vi "pcbAlignment.vi"() -> ()   [LabVIEW 2015]
uses:
  GlobalPath.vi
  GlobalData.vi
  GlobalVi.vi
panel:
  out "appended path":path
  out "appended path":path
  out "Execution:State":T1(ring)
  out "rasnik program 2":bool
  out "Open Program 2":bool
  in  "Open Program 6":bool
  out "Mapping file":string
  in  "?":bool
  in  "visual 4":bool caption="Close the PCB gaps to not lose vacuum pressure"
  in  "Open Program 5":bool
  in  "Open Program 4":bool
  in  "Done with vacuum test?":bool
  in  "c-ccd 9":bool caption="Place the movement arch away from the table"
  in  "c-ccd 8":bool caption="Release the movement arch from the stiffback"
  in  "c-ccd 7":bool caption="Lower the stiffback on the table"
  in  "c-ccd 6":bool caption="Move the stiffback over the table"
  in  "Open Program 3":bool
  out "PanelName":string
  in  "rasnik program":bool
  in  "Done with PCB testing?":bool
  in  "Open Program":bool
  in  "c-ccd 4":bool caption="Remove the 10 reference pins"
  in  "visual 3":bool caption="Turn vacuum on for PCB blocking"
  in  "Done?":bool
  in  "visual 2":bool caption="Position the 10 reference pins for the PCB alignment"
  # "PCB alignment on table/stiffback"
  # "Vacuum testing"
  # "Open the pressure monitoring program and let it run on the background"
  # "and press \"Start\" to start the pressure recording"
  # "Check the PCB vacuum"
  # "choose the date and press ok to make sure the pressure levels are alright"
  # "Rasnik mask reading from C-CCDs"
  # "The PCB on the table/stiffback will be read through the appropriate vi program"
  # "Post-alignment"
  # "PCB testing"
  # "At this point, the PCB on the table/stiffback will be tested in the appropriate vi program"
  # "PCB MAPPING"
  # "IN CASE OF PCB QUALITY PROBLEMS:\n(only press if need of PCB substitution)"
  # "FRAME/COOLING BAR MAPPING"
  # "Loading the raw file to the database:\nGo to the Database, select the tab \"PCB\" and then for each PCB (cross-check the positions from the \"Position\" selection within each PCB tab) click on \"Load Raw\"\nand choose the appropritate file to load ---->\nClick on \"Add/Update Entry\""
  # "(If the database window is closed, then click here  -->                 and load the correct panel this way: Add>Add then from the list choose \"Readout\" and then Start\n                                                                                                                                                                                                                     Choose the correct ID and click \"Start building panel\")"
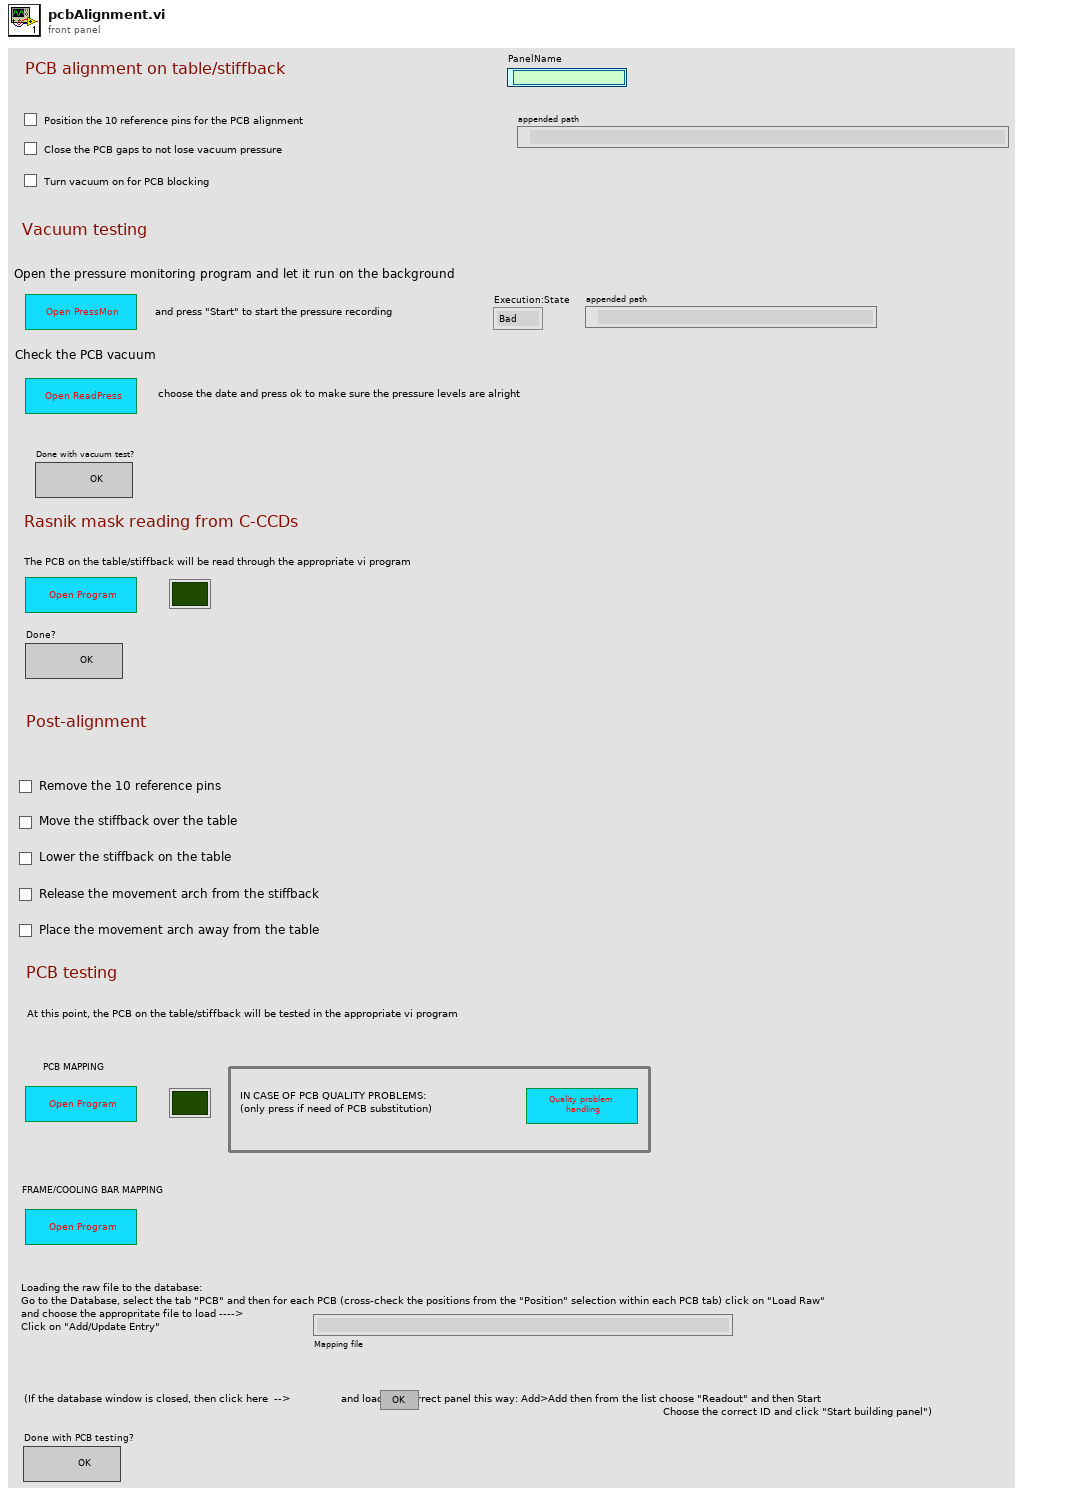
[diagram p1: front panel]
types:
  T1 = enum32{"Bad", "Idle", "Run top level", "Running"}
  T2 = enum16{"open", "replace", "create", "open or create", "replace or create", "replace or create with confirmation"}
  T3 = enum8{"Enabled", "Disabled", "Disabled and Grayed Out"}
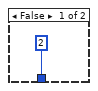
[diagram p4: hidden frame]
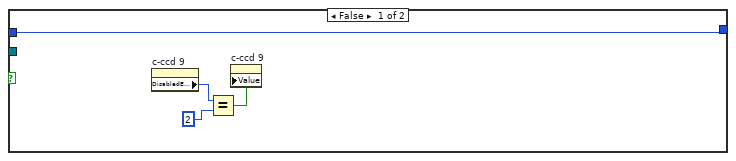
[diagram p8: hidden frame]
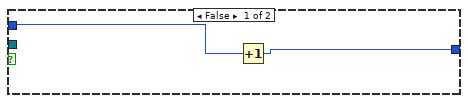
[diagram p9: hidden frame]
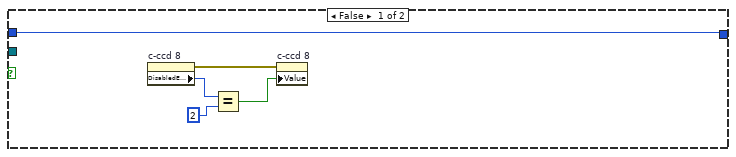
[diagram p10: hidden frame]
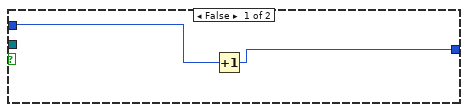
[diagram p11: hidden frame]
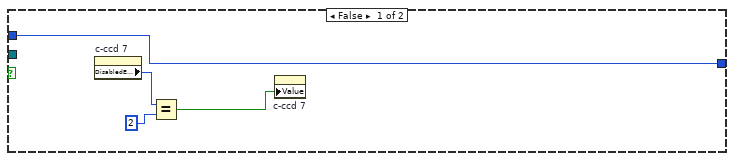
[diagram p12: hidden frame]
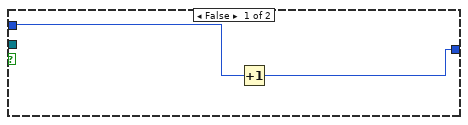
[diagram p13: hidden frame]
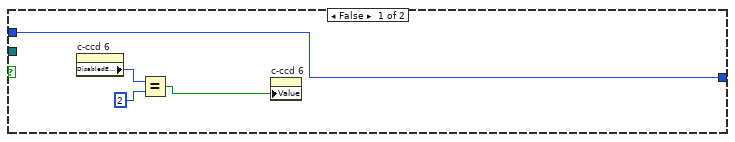
[diagram p14: hidden frame]
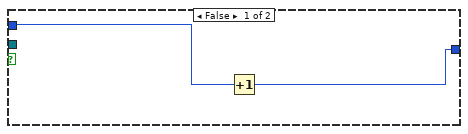
[diagram p15: hidden frame]
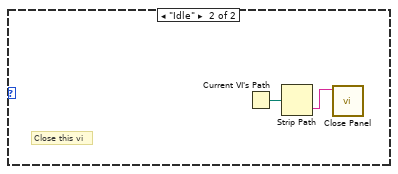
[diagram p19: hidden frame]
diagram:
  n1 = flat-sequence {
    tunnel: [w13] -> w10
    tunnel: [w12] -> w9
    tunnel: w10 -> [w73]
    tunnel: w9 -> [w72]
    tunnel: [w73] -> w8
    tunnel: [w72] -> w7
    tunnel: w8 -> [w411]
    tunnel: w7 -> [w410]
    tunnel: [w404] -> w6
    tunnel: [w409] -> w5
    tunnel: w6 -> [w513]
    tunnel: w5 -> [w524]
    tunnel: [w524] -> w4
    tunnel: [w512] -> w2
    tunnel: w4 -> [w539]
    tunnel: [w539] -> w3
    tunnel: w2 -> [w535]
    tunnel: [w534] -> w1
    tunnel: w3 -> [_]
    tunnel: w1 -> [_]
    frame #0 {
      n2 = flat-sequence {
        tunnel: [w26] -> w14
        tunnel: [w25] -> w11
        tunnel: w14 -> [w55]
        tunnel: [w54] -> w13
        tunnel: [w53] -> w12
        tunnel: w11 -> [w52]
        frame #0 {
          n3 = global read "GlobalData.vi" "PanelName"() -> (w20:string)
          n4 = global read "GlobalPath.vi" "LogFilesDir"() -> (w18:path)
          n5 = global read "GlobalData.vi" "Stage"() -> (w17:string)
          n6 = Empty String/Path?(string/path=w17) -> (empty?=w19:bool)
          n7 = Empty String/Path?(string/path=w20) -> (empty?=w21:bool)
          n8 = case shown="True" w19 {
            tunnel: w18 -> [_ w38]
            tunnel: [w32 w33] -> w16
            tunnel: w17 -> [w32 _]
            frame False {
            }
            frame True {
              n9 = Build Path(base path=w38, name or relative path="Stage.log") -> (appended path=w37:path)
              n10 = Open/Create/Replace File(file path (use dialog)=w37) -> (refnum out=w34:refnum<file>, error out=w35:errorcluster)  [unwired: 5 in, 1 out]
              n11 = Read from Text File(file (use dialog)=w34, error in=w35) -> (text=w33:string)  [unwired: 2 in, 3 out]
              n12 = global write "GlobalData.vi" "Stage"(w33) -> ()
            }
          }
          n13 = case shown="True" w21 {
            tunnel: w18 -> [_ w45]
            tunnel: [w39 w40] -> w15
            tunnel: w20 -> [w39 _]
            frame False {
            }
            frame True {
              n14 = Build Path(base path=w45, name or relative path="PanelName.log") -> (appended path=w44:path)
              n15 = Open/Create/Replace File(file path (use dialog)=w44) -> (refnum out=w41:refnum<file>, error out=w42:errorcluster)  [unwired: 5 in, 1 out]
              n16 = Read from Text File(file (use dialog)=w41, error in=w42) -> (text=w40:string)  [unwired: 2 in, 3 out]
              n17 = global write "GlobalData.vi" "PanelName"(w40) -> ()
            }
          }
          "PanelName" <- w15
          n18 = Equal?(x=w16, y="Stiffback") -> (x = y?=w23:bool)
          n19 = Build Path(base path=w18, name or relative path=w15) -> (appended path=w31:path)
          "appended path" <- w31
          n20 = case shown="True" w23 {
            tunnel: [2 0] -> w22
            frame False {
            }
            frame True {
            }
          }
          n21 = property on="c-ccd 6" class="Bool (strict)"("DisabledEnum"=w22) -> ()  [unwired: 2 in, 2 out]
          n22 = property on="c-ccd 8" class="Bool (strict)"("DisabledEnum"=w22) -> ()  [unwired: 2 in, 2 out]
          n23 = property on="c-ccd 9" class="Bool (strict)"("DisabledEnum"=w22) -> ()  [unwired: 2 in, 2 out]
          n24 = property on="c-ccd 7" class="Bool (strict)"("DisabledEnum"=w22) -> ()  [unwired: 2 in, 2 out]
          n25 = Open/Create/Replace File(file path (use dialog)=w31, operation (0:open)=T2."open") -> (refnum out=w28:refnum<file>, error out=w27:errorcluster)  [unwired: 4 in, 1 out]
          n26 = Set File Position(refnum=w28, from (0:start)=enum16{"start", "end", "current"}."end", error in=w27) -> (refnum out=w26:refnum<file>, error out=w25:errorcluster)  [unwired: 1 in]
        }
        frame #1 {
          w48 = "\r"
          n27 = Get Date/Time In Seconds() -> (seconds since 1Jan1904=w51:timestamp)
          n28 = global read "GlobalData.vi" "Stage"() -> (w50:string)
          n29 = Format Date/Time String(seconds (now)=w51) -> (date/time string=w57:string)  [unwired: 2 in]
          n30 = Concatenate Strings(w48, w57, "\t", " PCB ALIGNMENT ", w50, ": ", w48) -> (w56:string)
          n31 = Write to Text File(file (use dialog)=w55, text=w56, error in=w52) -> (refnum out=w54:refnum<file>, error out=w53:errorcluster)  [unwired: 1 in, 1 out]
        }
      }
    }
    frame #1 {
      n32 = while {
        tunnel: w73 -> [w81]
        shift-right: [w132] -> _
        shift-left: 0 -> [w130]
        shift-right: [w127] -> _
        shift-left: 0 -> [w123]
        shift-right: [w114] -> _
        shift-left: 0 -> [w119]
        shift-right: [w115] -> _
        shift-left: 0 -> [w116]
        shift-right: [w109] -> _
        shift-left: 0 -> [w110]
        shift-right: [w104] -> _
        shift-left: 0 -> [w106]
        shift-right: [w92] -> _
        shift-left: 0 -> [w99]
        shift-right: [w93] -> _
        shift-left: 0 -> [w98]
        shift-right: [w94] -> _
        shift-left: 0 -> [w97]
        shift-right: [w95] -> _
        shift-left: 0 -> [w96]
        shift-right: [w84] -> _
        shift-left: 0 -> [w85]
        shift-right: [w79] -> _
        shift-left: 0 -> [w82]
        stop <- w134 stop-if-true
        n33 = Compound Arithmetic op=AND("visual 2", "visual 3", "Open Program 4", "Done?", "c-ccd 4", "visual 4", "Open Program 6", "c-ccd 6", "c-ccd 7", "c-ccd 8", "c-ccd 9") -> (w134:bool)
        n34 = Equal To 0?(x=w82) -> (x = 0?=w83:bool)
        n35 = Equal To 0?(x=w119) -> (x = 0?=w122:bool)
        n36 = Equal To 0?(x=w106) -> (x = 0?=w108:bool)
        n37 = Equal To 0?(x=w99) -> (x = 0?=w103:bool)
        n38 = Equal To 0?(x=w97) -> (x = 0?=w101:bool)
        n39 = Equal To 0?(x=w96) -> (x = 0?=w100:bool)
        n40 = Equal To 0?(x=w130) -> (x = 0?=w129:bool)
        n41 = Equal To 0?(x=w98) -> (x = 0?=w102:bool)
        n42 = Equal To 0?(x=w110) -> (x = 0?=w113:bool)
        n43 = Equal To 0?(x=w116) -> (x = 0?=w118:bool)
        n44 = Equal To 0?(x=w123) -> (x = 0?=w126:bool)
        n45 = Wait (ms)(milliseconds to wait=u32 50) -> ()  [unwired: 1 out]
        n46 = And(x="Open Program 6", y=w83) -> (x .and. y?=w80:bool)
        n47 = And(x="rasnik program", y=w122) -> (x .and. y?=w120:bool)
        n48 = And(x="c-ccd 4", y=w108) -> (x .and. y?=w107:bool)
        n49 = And(x="c-ccd 6", y=w103) -> (x .and. y?=w88:bool)
        n50 = And(x="c-ccd 8", y=w101) -> (x .and. y?=w90:bool)
        n51 = And(x="c-ccd 9", y=w100) -> (x .and. y?=w91:bool)
        n52 = And(x="visual 2", y=w129) -> (x .and. y?=w128:bool)
        n53 = And(x="c-ccd 7", y=w102) -> (x .and. y?=w89:bool)
        n54 = And(x="Done?", y=w113) -> (x .and. y?=w111:bool)
        n55 = And(x="Open Program 4", y=w118) -> (x .and. y?=w117:bool)
        n56 = And(x="visual 3", y=w126) -> (x .and. y?=w124:bool)
        n57 = case shown="True" w111 {
          tunnel: w81 -> [_ w290]
          tunnel: [w286 w289] -> w109
          tunnel: w110 -> [w286 w288]
          frame False {
          }
          frame True {
            n58 = flat-sequence {
              tunnel: w290 -> [w293]
              tunnel: [w292] -> w291
              tunnel: w288 -> [w292]
              tunnel: w291 -> [w297]
              tunnel: [w298] -> w287
              tunnel: [w299] -> w289
              tunnel: w287 -> [w299]
              frame #0 {
                n59 = Concatenate Strings("Done with Rasmask reading", "\r") -> (w296:string)
                n60 = Write to Text File(file (use dialog)=w293, text=w296) -> ()  [unwired: 2 in, 3 out]
              }
              frame #1 {
                n61 = Increment(x=w297) -> (x+1=w298:i32)
              }
              frame #2 {
                n62 = while {
                  stop <- TRUE stop-if-true
                  n63 = property on="Open Program 3" class="Bool (strict)"() -> ("Value"=w301:bool)  [unwired: 2 in, 2 out]
                  n64 = Wait (ms)(milliseconds to wait=10000) -> ()  [unwired: 1 out]
                  n65 = Equal?(x=w301, y=TRUE) -> (x = y?=w303:bool)
                  n66 = case shown="True" w303 {
                    frame False {
                    }
                    frame True {
                      # "Automatically open the QualityProblemHandling.vi and close the current vi once done"
                      n67 = global read "GlobalPath.vi" "ViDir"() -> (w307:path)
                      n68 = call "OpenNRun.vi"("VI name"="QualityProblemHandling.vi", "ViDirPath"=w307) -> ("Execution:State"=w306:T1)
                      n69 = case shown="\"Bad\", Default" w306 {
                        frame "Bad", Default {
                          n70 = flat-sequence {
                            tunnel: [w309] -> w308
                            tunnel: w308 -> [w312]
                            frame #0 {
                              n71 = call "Display Message to User5"() -> ("error out"=w309:errorcluster)  [unwired: 10 in, 1 out]
                            }
                            frame #1 {
                              n72 = Current VI's Path() -> (path=w310:path)
                              n73 = Open VI Reference(vi path=w310, error in (no error)=w312) -> (vi reference=w315:refnum<vi>, error out=w314:errorcluster)  [unwired: 4 in]
                              n74 = global read "GlobalPath.vi" "ViDir"() -> (w311:path)
                              n75 = property class="VI"(reference=w315, error in=w314) -> ("Name"=w313:string)  [unwired: 2 out]
                              n76 = call "OpenNRun.vi"("VI name"=w313, "ViDirPath"=w311) -> ()  [unwired: 1 out]
                            }
                          }
                        }
                        frame "Idle" {
                          # "Close this vi"
                          n77 = Current VI's Path() -> (path=w317:path)
                          n78 = Strip Path(path=w317) -> (name=w316:string)  [unwired: 1 out]
                          n79 = call <vilib>:"Close Panel.vi"("VI name"=w316) -> ()  [unwired: 10 in, 1 out]
                        }
                      }
                    }
                  }
                }
              }
            }
          }
        }
        n80 = case shown="True" w80 {
          tunnel: w81 -> [_ w143]
          tunnel: [w135 w142] -> w79
          tunnel: w82 -> [w135 w141]
          frame False {
          }
          frame True {
            n81 = flat-sequence {
              tunnel: w143 -> [w145]
              tunnel: [w146] -> w144
              tunnel: w141 -> [w146]
              tunnel: [w145] -> w138
              tunnel: w144 -> [w154]
              tunnel: [w155] -> w140
              tunnel: w138 -> [w153]
              tunnel: [w153] -> w136
              tunnel: w140 -> [w162]
              tunnel: [w162] -> w139
              tunnel: [w161] -> w137
              tunnel: w136 -> [w161]
              tunnel: [w168] -> w142
              tunnel: w139 -> [w168]
              tunnel: w137 -> [w164]
              frame #0 {
                n82 = Concatenate Strings("Calling readpress.vi", "\r") -> (w149:string)
                n83 = Write to Text File(file (use dialog)=w145, text=w149) -> ()  [unwired: 2 in, 3 out]
              }
              frame #1 {
                n84 = global read "GlobalPath.vi" "ViDir"() -> (w152:path)
                n85 = Increment(x=w154) -> (x+1=w155:i32)
                n86 = call "OpenNRun.vi"("VI name"="readPress.vi", "ViDirPath"=w152) -> ("Execution:State"=w150:T1)
                n87 = case shown="\"Bad\", Default" w150 {
                  frame "Bad", Default {
                    n88 = flat-sequence {
                      frame #0 {
                        n89 = call "Display Message to User9"() -> ()  [unwired: 10 in, 2 out]
                      }
                      frame #1 {
                        n90 = Current VI's Path() -> (path=w156:path)
                        n91 = Open VI Reference(vi path=w156) -> (vi reference=w160:refnum<vi>, error out=w159:errorcluster)  [unwired: 5 in]
                        n92 = global read "GlobalPath.vi" "ViDir"() -> (w158:path)
                        n93 = property class="VI"(reference=w160, error in=w159) -> ("Name"=w157:string)  [unwired: 2 out]
                        n94 = call "OpenNRun.vi"("VI name"=w157, "ViDirPath"=w158) -> ()  [unwired: 1 out]
                      }
                    }
                  }
                  frame "Idle" {
                  }
                }
              }
              frame #2 {
                n95 = while {
                  stop <- "Done with vacuum test?" stop-if-true
                }
              }
              frame #3 {
                n96 = Concatenate Strings("Done with reading pressure", "\r") -> (w167:string)
                n97 = Write to Text File(file (use dialog)=w164, text=w167) -> ()  [unwired: 2 in, 3 out]
              }
            }
          }
        }
        n98 = case shown="True" w88 {
          tunnel: w99 -> [w251 w260]
          tunnel: w81 -> [_ w259]
          tunnel: [w251 w258] -> w92
          frame False {
            n99 = property on="c-ccd 6" class="Bool (strict)"() -> ("DisabledEnum"=w253:T3)  [unwired: 2 in, 2 out]
            n100 = Equal?(x=w253, y=2) -> (x = y?=w252:bool)
            n101 = property on="c-ccd 6" class="Bool (strict)"("Value"=w252) -> ()  [unwired: 2 in, 2 out]
          }
          frame True {
            n102 = property on="c-ccd 6" class="Bool (strict)"() -> ("DisabledEnum"=w256:T3)  [unwired: 2 in, 2 out]
            n103 = Equal?(x=w256, y=0) -> (x = y?=w255:bool)
            n104 = case shown="True" w255 {
              tunnel: w259 -> [_ w265]
              tunnel: [w261 w264] -> w258
              tunnel: w260 -> [w262 w263]
              frame False {
                n105 = Increment(x=w262) -> (x+1=w261:i32)
              }
              frame True {
                n106 = flat-sequence {
                  tunnel: w265 -> [w268]
                  tunnel: [w267] -> w266
                  tunnel: w263 -> [w267]
                  tunnel: w266 -> [w272]
                  tunnel: [w273] -> w264
                  frame #0 {
                    n107 = Concatenate Strings("Stiffback moved over table", "\r") -> (w271:string)
                    n108 = Write to Text File(file (use dialog)=w268, text=w271) -> ()  [unwired: 2 in, 3 out]
                  }
                  frame #1 {
                    n109 = Increment(x=w272) -> (x+1=w273:i32)
                  }
                }
              }
            }
          }
        }
        n110 = case shown="True" w89 {
          tunnel: w81 -> [_ w237]
          tunnel: w98 -> [w228 w236]
          tunnel: [w228 w235] -> w93
          frame False {
            n111 = property on="c-ccd 7" class="Bool (strict)"() -> ("DisabledEnum"=w230:T3)  [unwired: 2 in, 2 out]
            n112 = Equal?(x=w230, y=2) -> (x = y?=w229:bool)
            n113 = property on="c-ccd 7" class="Bool (strict)"("Value"=w229) -> ()  [unwired: 2 in, 2 out]
          }
          frame True {
            n114 = property on="c-ccd 7" class="Bool (strict)"() -> ("DisabledEnum"=w233:T3)  [unwired: 2 in, 2 out]
            n115 = Equal?(x=w233, y=0) -> (x = y?=w232:bool)
            n116 = case shown="True" w232 {
              tunnel: w237 -> [_ w242]
              tunnel: [w238 w241] -> w235
              tunnel: w236 -> [w239 w240]
              frame False {
                n117 = Increment(x=w239) -> (x+1=w238:i32)
              }
              frame True {
                n118 = flat-sequence {
                  tunnel: w242 -> [w245]
                  tunnel: [w244] -> w243
                  tunnel: w240 -> [w244]
                  tunnel: w243 -> [w249]
                  tunnel: [w250] -> w241
                  frame #0 {
                    n119 = Concatenate Strings("Stiffback lowered on table", "\r") -> (w248:string)
                    n120 = Write to Text File(file (use dialog)=w245, text=w248) -> ()  [unwired: 2 in, 3 out]
                  }
                  frame #1 {
                    n121 = Increment(x=w249) -> (x+1=w250:i32)
                  }
                }
              }
            }
          }
        }
        n122 = case shown="True" w90 {
          tunnel: w81 -> [_ w214]
          tunnel: w97 -> [w204 w213]
          tunnel: [w204 w212] -> w94
          frame False {
            n123 = property on="c-ccd 8" class="Bool (strict)"() -> (error out=w208:errorcluster, "DisabledEnum"=w206:T3)  [unwired: 2 in, 1 out]
            n124 = Equal?(x=w206, y=2) -> (x = y?=w205:bool)
            n125 = property on="c-ccd 8" class="Bool (strict)"(error in=w208, "Value"=w205) -> ()  [unwired: 1 in, 2 out]
          }
          frame True {
            n126 = property on="c-ccd 8" class="Bool (strict)"() -> ("DisabledEnum"=w210:T3)  [unwired: 2 in, 2 out]
            n127 = Equal?(x=w210, y=0) -> (x = y?=w209:bool)
            n128 = case shown="True" w209 {
              tunnel: w214 -> [_ w219]
              tunnel: [w215 w218] -> w212
              tunnel: w213 -> [w216 w217]
              frame False {
                n129 = Increment(x=w216) -> (x+1=w215:i32)
              }
              frame True {
                n130 = flat-sequence {
                  tunnel: w219 -> [w222]
                  tunnel: [w221] -> w220
                  tunnel: w217 -> [w221]
                  tunnel: w220 -> [w226]
                  tunnel: [w227] -> w218
                  frame #0 {
                    n131 = Concatenate Strings("Arch released", "\r") -> (w225:string)
                    n132 = Write to Text File(file (use dialog)=w222, text=w225) -> ()  [unwired: 2 in, 3 out]
                  }
                  frame #1 {
                    n133 = Increment(x=w226) -> (x+1=w227:i32)
                  }
                }
              }
            }
          }
        }
        n134 = case shown="True" w91 {
          tunnel: w81 -> [_ w186]
          tunnel: w96 -> [w181 w187]
          tunnel: [w181 w185] -> w95
          frame False {
            n135 = property on="c-ccd 9" class="Bool (strict)"() -> ("DisabledEnum"=w183:T3)  [unwired: 2 in, 2 out]
            n136 = Equal?(x=w183, y=2) -> (x = y?=w182:bool)
            n137 = property on="c-ccd 9" class="Bool (strict)"("Value"=w182) -> ()  [unwired: 2 in, 2 out]
          }
          frame True {
            n138 = property on="c-ccd 9" class="Bool (strict)"() -> ("DisabledEnum"=w189:T3)  [unwired: 2 in, 2 out]
            n139 = Equal?(x=w189, y=0) -> (x = y?=w188:bool)
            n140 = case shown="True" w188 {
              tunnel: w186 -> [_ w195]
              tunnel: [w191 w194] -> w185
              tunnel: w187 -> [w192 w193]
              frame False {
                n141 = Increment(x=w192) -> (x+1=w191:i32)
              }
              frame True {
                n142 = flat-sequence {
                  tunnel: w195 -> [w198]
                  tunnel: [w197] -> w196
                  tunnel: w193 -> [w197]
                  tunnel: w196 -> [w202]
                  tunnel: [w203] -> w194
                  frame #0 {
                    n143 = Concatenate Strings("Arch moved away", "\r") -> (w201:string)
                    n144 = Write to Text File(file (use dialog)=w198, text=w201) -> ()  [unwired: 2 in, 3 out]
                  }
                  frame #1 {
                    n145 = Increment(x=w202) -> (x+1=w203:i32)
                  }
                }
              }
            }
          }
        }
        n146 = case shown="True" w117 {
          tunnel: w81 -> [_ w326]
          tunnel: [w318 w325] -> w115
          tunnel: w116 -> [w318 w324]
          frame False {
          }
          frame True {
            n147 = flat-sequence {
              tunnel: w326 -> [w328]
              tunnel: [w329] -> w327
              tunnel: w324 -> [w329]
              tunnel: [w328] -> w321
              tunnel: w327 -> [w341]
              tunnel: [w342] -> w323
              tunnel: w321 -> [w340]
              tunnel: [w340] -> w319
              tunnel: w323 -> [w352]
              tunnel: [w352] -> w322
              tunnel: [w351] -> w320
              tunnel: w319 -> [w351]
              tunnel: [w357] -> w325
              tunnel: w322 -> [w357]
              tunnel: w320 -> [w353]
              frame #0 {
                n148 = Concatenate Strings("Calling pressmon.vi", "\r") -> (w332:string)
                n149 = Write to Text File(file (use dialog)=w328, text=w332) -> ()  [unwired: 2 in, 3 out]
              }
              frame #1 {
                w336 = "pressmon.vi"
                n150 = global read "GlobalPath.vi" "ViDir"() -> (w334:path)
                n151 = Increment(x=w341) -> (x+1=w342:i32)
                n152 = Build Path(base path=path "/home/atlas/Micromegas/interface" ("ViDir"), name or relative path=w336) -> (appended path=w337:path)
                "appended path" <- w337
                n153 = Open VI Reference(vi path=w337) -> (vi reference=w338:refnum<vi>, error out=w339:errorcluster)  [unwired: 5 in]
                n154 = property class="VI"(reference=w338, error in=w339) -> ("Exec.State"=w335:T1)  [unwired: 2 out]
                "Execution:State" <- w335
                n155 = case shown="\"Bad\", Default" w335 {
                  tunnel: w336 -> [_ w345 _ _]
                  tunnel: w334 -> [_ w343 _ _]
                  frame "Bad", Default {
                  }
                  frame "Idle" {
                    n156 = call "OpenNRun.vi"("VI name"=w345, "ViDirPath"=w343) -> ("Execution:State"=w344:T1)
                    n157 = case shown="\"Bad\", Default" w344 {
                      frame "Bad", Default {
                        n158 = flat-sequence {
                          frame #0 {
                            n159 = call "Display Message to User6"() -> ()  [unwired: 10 in, 2 out]
                          }
                          frame #1 {
                            n160 = Current VI's Path() -> (path=w346:path)
                            n161 = Open VI Reference(vi path=w346) -> (vi reference=w350:refnum<vi>, error out=w349:errorcluster)  [unwired: 5 in]
                            n162 = global read "GlobalPath.vi" "ViDir"() -> (w348:path)
                            n163 = property class="VI"(reference=w350, error in=w349) -> ("Name"=w347:string)  [unwired: 2 out]
                            n164 = call "OpenNRun.vi"("VI name"=w347, "ViDirPath"=w348) -> ()  [unwired: 1 out]
                          }
                        }
                      }
                      frame "Idle" {
                      }
                    }
                  }
                  frame "Run top level" {
                  }
                  frame "Running" {
                  }
                }
              }
              frame #2 {
              }
              frame #3 {
                n165 = Concatenate Strings("Done with pressure monitoring", "\r") -> (w356:string)
                n166 = Write to Text File(file (use dialog)=w353, text=w356) -> ()  [unwired: 2 in, 3 out]
              }
            }
          }
        }
        n167 = case shown="True" w107 {
          tunnel: w81 -> [_ w277]
          tunnel: [w274 w276] -> w104
          tunnel: w106 -> [w274 w275]
          frame False {
          }
          frame True {
            n168 = flat-sequence {
              tunnel: w277 -> [w280]
              tunnel: [w279] -> w278
              tunnel: w275 -> [w279]
              tunnel: w278 -> [w284]
              tunnel: [w285] -> w276
              frame #0 {
                n169 = Concatenate Strings("Reference pins removed", "\r") -> (w283:string)
                n170 = Write to Text File(file (use dialog)=w280, text=w283) -> ()  [unwired: 2 in, 3 out]
              }
              frame #1 {
                n171 = Increment(x=w284) -> (x+1=w285:i32)
              }
            }
          }
        }
        n172 = case shown="True" w120 {
          tunnel: w81 -> [_ w361]
          tunnel: [w358 w359] -> w114
          tunnel: w119 -> [w358 w360]
          frame False {
          }
          frame True {
            n173 = flat-sequence {
              tunnel: w361 -> [w364]
              tunnel: [w363] -> w362
              tunnel: w360 -> [w363]
              tunnel: w362 -> [w371]
              tunnel: [w372] -> w359
              frame #0 {
                n174 = Concatenate Strings("Calling Rasnik.vi", "\r") -> (w367:string)
                n175 = Write to Text File(file (use dialog)=w364, text=w367) -> ()  [unwired: 2 in, 3 out]
              }
              frame #1 {
                n176 = global read "GlobalPath.vi" "ViDir"() -> (w368:path)
                n177 = Increment(x=w371) -> (x+1=w372:i32)
                n178 = call "OpenNRun.vi"("VI name"="Rasnik.vi", "ViDirPath"=w368) -> ("Execution:State"=w369:T1)
                n179 = case shown="\"Bad\", Default" w369 {
                  frame "Bad", Default {
                    n180 = flat-sequence {
                      frame #0 {
                        n181 = call "Display Message to User3"() -> ()  [unwired: 10 in, 2 out]
                      }
                      frame #1 {
                        n182 = Current VI's Path() -> (path=w373:path)
                        n183 = Open VI Reference(vi path=w373) -> (vi reference=w377:refnum<vi>, error out=w376:errorcluster)  [unwired: 5 in]
                        n184 = global read "GlobalPath.vi" "ViDir"() -> (w375:path)
                        n185 = property class="VI"(reference=w377, error in=w376) -> ("Name"=w374:string)  [unwired: 2 out]
                        n186 = call "OpenNRun.vi"("VI name"=w374, "ViDirPath"=w375) -> ()  [unwired: 1 out]
                      }
                    }
                  }
                  frame "Idle" {
                  }
                }
              }
            }
          }
        }
        n187 = case shown="True" w128 {
          tunnel: w81 -> [_ w394]
          tunnel: w130 -> [w390 w393]
          tunnel: [w390 w391] -> w132
          frame False {
          }
          frame True {
            n188 = flat-sequence {
              tunnel: w394 -> [w396]
              tunnel: w393 -> [w395]
              tunnel: [w395] -> w392
              tunnel: w392 -> [w401]
              tunnel: [w400] -> w391
              frame #0 {
                n189 = Concatenate Strings("10 reference pins positioned", "\r") -> (w399:string)
                n190 = Write to Text File(file (use dialog)=w396, text=w399) -> ()  [unwired: 2 in, 3 out]
              }
              frame #1 {
                n191 = Increment(x=w401) -> (x+1=w400:i32)
              }
            }
          }
        }
        n192 = case shown="True" "visual 4" {
          tunnel: w81 -> [_ w172]
          tunnel: [w169 w171] -> w84
          tunnel: w85 -> [w169 w170]
          frame False {
          }
          frame True {
            n193 = flat-sequence {
              tunnel: w172 -> [w175]
              tunnel: [w174] -> w173
              tunnel: w170 -> [w174]
              tunnel: w173 -> [w179]
              tunnel: [w180] -> w171
              frame #0 {
                n194 = Concatenate Strings("Closing gaps", "\r") -> (w178:string)
                n195 = Write to Text File(file (use dialog)=w175, text=w178) -> ()  [unwired: 2 in, 3 out]
              }
              frame #1 {
                n196 = Increment(x=w179) -> (x+1=w180:i32)
              }
            }
          }
        }
        n197 = case shown="True" w124 {
          tunnel: w81 -> [_ w381]
          tunnel: [w378 w380] -> w127
          tunnel: w123 -> [w378 w379]
          frame False {
          }
          frame True {
            n198 = flat-sequence {
              tunnel: w381 -> [w384]
              tunnel: [w383] -> w382
              tunnel: w379 -> [w383]
              tunnel: w382 -> [w388]
              tunnel: [w389] -> w380
              frame #0 {
                n199 = Concatenate Strings("Vacuum turned on for blocking", "\r") -> (w387:string)
                n200 = Write to Text File(file (use dialog)=w384, text=w387) -> ()  [unwired: 2 in, 3 out]
              }
              frame #1 {
                n201 = Increment(x=w388) -> (x+1=w389:i32)
              }
            }
          }
        }
        "rasnik program 2" <- "rasnik program"
      }
    }
    frame #2 {
      # "PCB testing"
      n202 = while {
        shift-right: [w436] -> w403
        shift-left: w410 -> [w435]
        stop <- "Open Program" stop-if-true
        n203 = case shown="True" "Open Program" {
          tunnel: [w437 w439] -> w436
          tunnel: w435 -> [w437 w442]
          frame False {
          }
          frame True {
            n204 = flat-sequence {
              tunnel: w442 -> [w444]
              tunnel: [w443] -> w438
              tunnel: [w463] -> w441
              tunnel: [w462] -> w440
              tunnel: w438 -> [w461]
              tunnel: w441 -> [w469]
              tunnel: w440 -> [w468]
              tunnel: [w467] -> w439
              frame #0 {
                n205 = global read "GlobalPath.vi" "ViDir"() -> (w447:path)
                n206 = call "OpenNRun.vi"("VI name"="map_trap_switch.vi", "ViDirPath"=w447) -> ("Execution:State"=w446:T1)
                n207 = case shown="\"Bad\", Default" w446 {
                  tunnel: [w450 w460] -> w443
                  tunnel: w444 -> [w449 w460]
                  frame "Bad", Default {
                    n208 = flat-sequence {
                      tunnel: w449 -> [w452]
                      tunnel: [w451] -> w448
                      tunnel: [w455] -> w450
                      tunnel: w448 -> [w453]
                      frame #0 {
                        n209 = call "Display Message to User"("error in (no error)"=w452) -> ("error out"=w451:errorcluster)  [unwired: 9 in, 1 out]
                      }
                      frame #1 {
                        n210 = Current VI's Path() -> (path=w454:path)
                        n211 = Open VI Reference(vi path=w454, error in (no error)=w453) -> (vi reference=w459:refnum<vi>, error out=w458:errorcluster)  [unwired: 4 in]
                        n212 = global read "GlobalPath.vi" "ViDir"() -> (w457:path)
                        n213 = property class="VI"(reference=w459, error in=w458) -> (error out=w455:errorcluster, "Name"=w456:string)  [unwired: 1 out]
                        n214 = call "OpenNRun.vi"("VI name"=w456, "ViDirPath"=w457) -> ()  [unwired: 1 out]
                      }
                    }
                  }
                  frame "Idle" {
                  }
                }
              }
              frame #1 {
                n215 = Open/Create/Replace File(file path (use dialog)=path "/home/atlas/Micromegas/M05Data/mapping/map_trap_filename.txt", error in=w461, operation (0:open)=T2."open") -> (refnum out=w463:refnum<file>, error out=w462:errorcluster)  [unwired: 3 in, 1 out]
                n216 = Read from Text File(file (use dialog)=w463, error in=w462) -> (text=→"Mapping file":string)  [unwired: 2 in, 3 out]
              }
              frame #2 {
                n217 = Close File(refnum=w469, error in=w468) -> (error out=w467:errorcluster)  [unwired: 1 out]
              }
            }
          }
        }
        "Open Program 2" <- "Open Program"
      }
      n218 = while {
        shift-right: [w414] -> w402
        shift-left: w403 -> [w413]
        stop <- "Open Program 5" stop-if-true
        n219 = case shown="True" "Open Program 5" {
          tunnel: [w415 w417] -> w414
          tunnel: w413 -> [w415 w416]
          frame False {
          }
          frame True {
            n220 = global read "GlobalPath.vi" "ViDir"() -> (w420:path)
            n221 = call "OpenNRun.vi"("VI name"="map_diag.vi", "ViDirPath"=w420) -> ("Execution:State"=w419:T1)
            n222 = case shown="\"Bad\", Default" w419 {
              tunnel: [w423 w433] -> w417
              tunnel: w416 -> [w422 w433]
              frame "Bad", Default {
                n223 = flat-sequence {
                  tunnel: w422 -> [w425]
                  tunnel: [w424] -> w421
                  tunnel: [w428] -> w423
                  tunnel: w421 -> [w426]
                  frame #0 {
                    n224 = call "Display Message to User7"("error in (no error)"=w425) -> ("error out"=w424:errorcluster)  [unwired: 9 in, 1 out]
                  }
                  frame #1 {
                    n225 = Current VI's Path() -> (path=w427:path)
                    n226 = Open VI Reference(vi path=w427, error in (no error)=w426) -> (vi reference=w432:refnum<vi>, error out=w431:errorcluster)  [unwired: 4 in]
                    n227 = global read "GlobalPath.vi" "ViDir"() -> (w430:path)
                    n228 = property class="VI"(reference=w432, error in=w431) -> (error out=w428:errorcluster, "Name"=w429:string)  [unwired: 1 out]
                    n229 = call "OpenNRun.vi"("VI name"=w429, "ViDirPath"=w430) -> ()  [unwired: 1 out]
                  }
                }
              }
              frame "Idle" {
              }
            }
          }
        }
      }
      n230 = property on="Open Program 3" class="Bool (strict)"() -> ("Value"=w408:bool)  [unwired: 2 in, 2 out]
      n231 = Equal?(x=w408, y=TRUE) -> (x = y?=w406:bool)
      n232 = while {
        tunnel: w411 -> [w496]
        tunnel: w402 -> [w495]
        tunnel: [w494] -> w409
        tunnel: [w493] -> w405
        stop <- w497 stop-if-true
        n233 = case shown="True" "?" {
          frame False {
          }
          frame True {
          }
        }
        n234 = case shown="True" "Done with PCB testing?" {
          selector: "Done with PCB testing?" -> [w501 w506]
          tunnel: [w501 w506] -> w497
          tunnel: w496 -> [w499 w505]
          tunnel: w495 -> [w500 w504]
          tunnel: [w500 w502] -> w493
          tunnel: [w499 w503] -> w494
          frame False {
          }
          frame True {
            n235 = Concatenate Strings("PCB tested", "\r") -> (w509:string)
            n236 = Write to Text File(file (use dialog)=w505, text=w509, error in=w504) -> (refnum out=w503:refnum<file>, error out=w502:errorcluster)  [unwired: 1 in, 1 out]
          }
        }
        n237 = Wait (ms)(milliseconds to wait=10000) -> ()  [unwired: 1 out]
      }
      n238 = case shown="True" w406 {
        tunnel: w405 -> [w470 w472]
        tunnel: [w470 w471] -> w404
        frame False {
        }
        frame True {
          # "Automatically open the QualityProblemHandling.vi and close the current vi once done"
          n239 = global read "GlobalPath.vi" "ViDir"() -> (w475:path)
          n240 = call "OpenNRun.vi"("VI name"="QualityProblemHandling.vi", "ViDirPath"=w475) -> ("Execution:State"=w474:T1)
          n241 = case shown="\"Bad\", Default" w474 {
            tunnel: w472 -> [w477 w488]
            tunnel: [w476 w488] -> w471
            frame "Bad", Default {
              n242 = flat-sequence {
                tunnel: [w480] -> w478
                tunnel: w477 -> [w479]
                tunnel: [w484] -> w476
                tunnel: w478 -> [w483]
                frame #0 {
                  n243 = call "Display Message to User4"("error in (no error)"=w479) -> ("error out"=w480:errorcluster)  [unwired: 9 in, 1 out]
                }
                frame #1 {
                  n244 = Current VI's Path() -> (path=w481:path)
                  n245 = Open VI Reference(vi path=w481, error in (no error)=w483) -> (vi reference=w487:refnum<vi>, error out=w486:errorcluster)  [unwired: 4 in]
                  n246 = global read "GlobalPath.vi" "ViDir"() -> (w482:path)
                  n247 = property class="VI"(reference=w487, error in=w486) -> (error out=w484:errorcluster, "Name"=w485:string)  [unwired: 1 out]
                  n248 = call "OpenNRun.vi"("VI name"=w485, "ViDirPath"=w482) -> ()  [unwired: 1 out]
                }
              }
            }
            frame "Idle" {
              # "Close this vi"
              n249 = Current VI's Path() -> (path=w490:path)
              n250 = Strip Path(path=w490) -> (name=w489:string)  [unwired: 1 out]
              n251 = call <vilib>:"Close Panel.vi"("VI name"=w489) -> ()  [unwired: 10 in, 1 out]
            }
          }
        }
      }
    }
    frame #3 {
      # "Setting the global vairables to show that this stage is done"
      n252 = global read "GlobalPath.vi" "LogFilesDir"() -> (w510:path)
      n253 = Build Path(base path=w510, name or relative path="GlobalVar_Recovery.txt") -> (appended path=w522:path)
      n254 = global read "GlobalData.vi" "Stage"() -> (w526:string)
      n255 = Open/Create/Replace File(file path (use dialog)=w522, error in=w513, operation (0:open)=T2."open") -> (refnum out=w518:refnum<file>, error out=w519:errorcluster)  [unwired: 3 in, 1 out]
      n256 = String Length(string=w526) -> (length=w529:i32)
      n257 = String Length(string="Table") -> (length=w528:i32)
      n258 = Set File Position(refnum=w518, from (0:start)=enum16{"start", "end", "current"}."end", error in=w519) -> (refnum out=w515:refnum<file>, error out=w514:errorcluster)  [unwired: 1 in]
      n259 = Equal?(x=w529, y=w528) -> (x = y?=w527:bool)
      n260 = case shown="False" w527 {
        tunnel: ["PCBalignStiff" "PCBalignTab"] -> w511
        frame False {
          n261 = global write "GlobalVi.vi" "PCBalignStiff"(TRUE) -> ()
        }
        frame True {
          n262 = global write "GlobalVi.vi" "PCBalignTab"(TRUE) -> ()
        }
      }
      n263 = Concatenate Strings(w511, "\r") -> (w517:string)
      n264 = Write to Text File(file (use dialog)=w515, text=w517, error in=w514) -> (error out=w512:errorcluster)  [unwired: 1 in, 2 out]
    }
    frame #4 {
      # "Automatically open the ViChoise and close the current vi once done"
      n265 = global read "GlobalPath.vi" "ViDir"() -> (w538:path)
      n266 = call "OpenNRun.vi"("VI name"="ViChoice.vi", "ViDirPath"=w538) -> ("Execution:State"=w537:T1)
      n267 = case shown="\"Bad\", Default" w537 {
        tunnel: [w542 w552] -> w534
        tunnel: w535 -> [w540 w553]
        frame "Bad", Default {
          n268 = flat-sequence {
            tunnel: w540 -> [w544]
            tunnel: [w543] -> w541
            tunnel: [w548] -> w542
            tunnel: w541 -> [w547]
            frame #0 {
              n269 = call "Display Message to User2"("error in (no error)"=w544) -> ("error out"=w543:errorcluster)  [unwired: 9 in, 1 out]
            }
            frame #1 {
              n270 = Current VI's Path() -> (path=w545:path)
              n271 = Open VI Reference(vi path=w545, error in (no error)=w547) -> (vi reference=w551:refnum<vi>, error out=w550:errorcluster)  [unwired: 4 in]
              n272 = global read "GlobalPath.vi" "ViDir"() -> (w546:path)
              n273 = property class="VI"(reference=w551, error in=w550) -> (error out=w548:errorcluster, "Name"=w549:string)  [unwired: 1 out]
              n274 = call "OpenNRun.vi"("VI name"=w549, "ViDirPath"=w546) -> ()  [unwired: 1 out]
            }
          }
        }
        frame "Idle" {
          # "Close this vi"
          n275 = Current VI's Path() -> (path=w555:path)
          n276 = Strip Path(path=w555) -> (name=w554:string)  [unwired: 1 out]
          n277 = call <vilib>:"Close Panel.vi"("error in (no error)"=w553, "VI name"=w554) -> ("error out"=w552:errorcluster)  [unwired: 9 in]
        }
      }
    }
    frame #5 {
    }
  }
